vi "Measurement.TestLauncher.vi"() -> ()   [LabVIEW 2017]
uses:
  Typedefs/Measurement.Type--Enum.ctl
  Measurement.Free/Measurement.Free.lvclass
  D:/upwork/Laser Measurement Tool/Laser/project/Subsystems/Measurement/Measurement.lvclass
  Measurement.Free.UI/Measurement.Free.UI.lvclass
  D:/upwork/Laser Measurement Tool/Laser/project/Subsystems/Measurement.UI/Measurement.UI.lvclass
  Measurement.Free/Typedefs/Configuration--Cluster.ctl
  Measurement.Free/Typedefs/Configuration.Hardware--Cluster.ctl
  Typedefs/Configuration.SMU--Cluster.ctl
  SMU/Typedefs/Configuration--Cluster.ctl
  Typedefs/Configuration.LIA--Cluster.ctl
  LIA/Typedefs/Configuration--Cluster.ctl
  Typedefs/Configuration.OPM--Cluster.ctl
  OPM/Typedefs/Configuration--Cluster.ctl
  Typedefs/Configuration.OPA--Cluster.ctl
  OPA/Typedefs/Configuration--Cluster.ctl
  Measurement.lvclass
  OPA/OPA.lvclass
  OPM/OPM.lvclass
  LIA/LIA.lvclass
  SMU/SMU.lvclass
  OPA.OrpheusHP/OPA.OrpheusHP.lvclass
  OPM.ThorlabsPM400/OPM.ThorlabsPM400.lvclass
panel:
  in  "Close":bool
  out "Measurements Tree":string(tree) caption="Chart A"
  in  "Add":bool
  in  "Remove":bool
  in  "Stop":bool
  in  "Start":bool
  in  "Measurement Parameters":T1(tab)
  in  "Accumulation":dbl=10.0 caption="Numeric"
  in  "Delay Time":dbl[unit]=0.5
  in  "Integration Time":dbl[unit]=3.0
  in  "Scan Resolution":dbl[unit]=2e-08
  in  "Number of Points":dbl caption="Numeric"
  in  "Stop Wavelength":dbl[unit]=1.0000000000000002e-06
  in  "Start Wavelength":dbl[unit]=6.000000000000001e-07
  in  "Sync":bool
  in  "Save":bool
  in  "Hardware Parameters":enum32{"Free"}(tab)
  in  "OPA Refresh List":bool
  in  "OPA Serial Number":string(combo)
  in  "OPM Refresh List":bool
  in  "OPM Simulated":bool
  in  "OPM Resource Name":string(combo)="USB0::0x1313::0x8075::P5001221::INSTR"
  in  "SMU Channel":string(combo)="A"
  in  "SMU Simulated":bool
  in  "SMU VISA Resource Name":refnum<visa-resource-name>="GPIB0::26::INSTR"
  in  "LIA Simulated":bool
  in  "LIA VISA Resource Name":refnum<visa-resource-name>="GPIB0::8::INSTR"
  out "Status":string
  out "Progress":u8(slide) scale=0.0..100.0
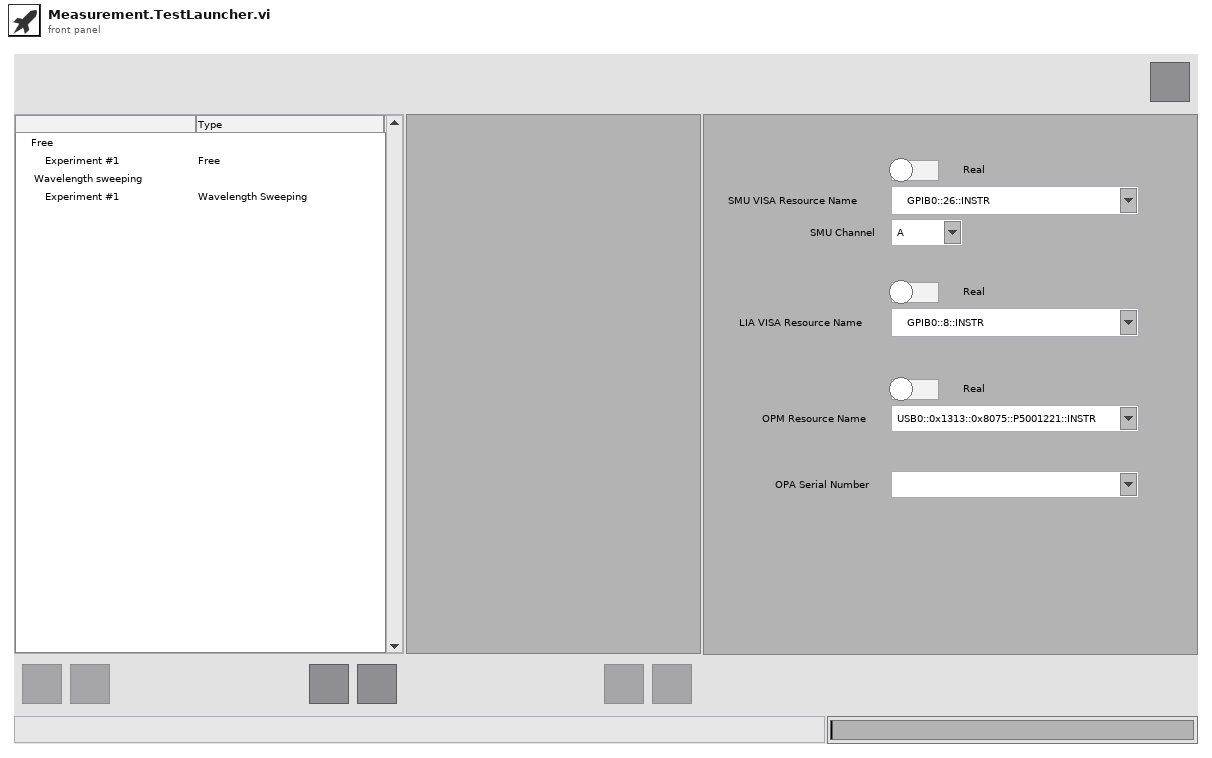
[diagram p1: front panel]
types:
  T1 = enum32{"Free", "Wavelength Sweeping", "Photocurrent mapping"}
  T2 = typedef "Measurement.lvclass/Measurement.Type--Enum.ctl" = enum16{"Free", "I/V Curve", "Wavelength sweeping", "Photocurrent mapping"}
  T3 = enum16{"Free", "I/V Curve", "Wavelength sweeping", "Photocurrent mapping"}
  T4 = enum8{"Enabled", "Disabled", "Disabled and Grayed Out"}
  T5 = typedef "LVPoint32TypeDef.ctl" = cluster{"Horizontal":i32, "Vertical":i32}
  T6 = typedef "Measurement.lvclass/Configuration.OPA--Cluster.ctl" = cluster{"Enable":bool, "OPA Model":string, "Configuration":T7}
  T7 = typedef "OPA.lvclass/Configuration--Cluster.ctl" = cluster{"Serial Number":string}
  T8 = typedef "Measurement.lvclass/Configuration.OPM--Cluster.ctl" = cluster{"Enable":bool, "OPM Model":string, "Configuration":T9}
  T9 = typedef "OPM.lvclass/Configuration--Cluster.ctl" = cluster{"VISA Resource":string}
  T10 = typedef "Measurement.lvclass/Configuration.LIA--Cluster.ctl" = cluster{"Enable":bool, "LIA Model":string, "Configuration":T11}
  T11 = typedef "LIA.lvclass/Configuration--Cluster.ctl" = cluster{"VISA Resource":string}
  T12 = typedef "Measurement.lvclass/Configuration.SMU--Cluster.ctl" = cluster{"Enable":bool, "SMU Model":string, "Configuration":T13}
  T13 = typedef "SMU.lvclass/Configuration--Cluster.ctl" = cluster{"VISA Resource":string, "Channel":string}
  T14 = typedef "Measurement.Free.lvclass/Configuration--Cluster.ctl" = cluster{"Measurement.Type":enum16{"Free", "I/V Curve", "Wavelength sweeping", "Photocurrent mapping"}, "Hardware":T15}
  T15 = typedef "Measurement.Free.lvclass/Configuration.Hardware--Cluster.ctl" = cluster{"SMU":T12, "LIA":T10, "OPM":T8, "OPA":T6}
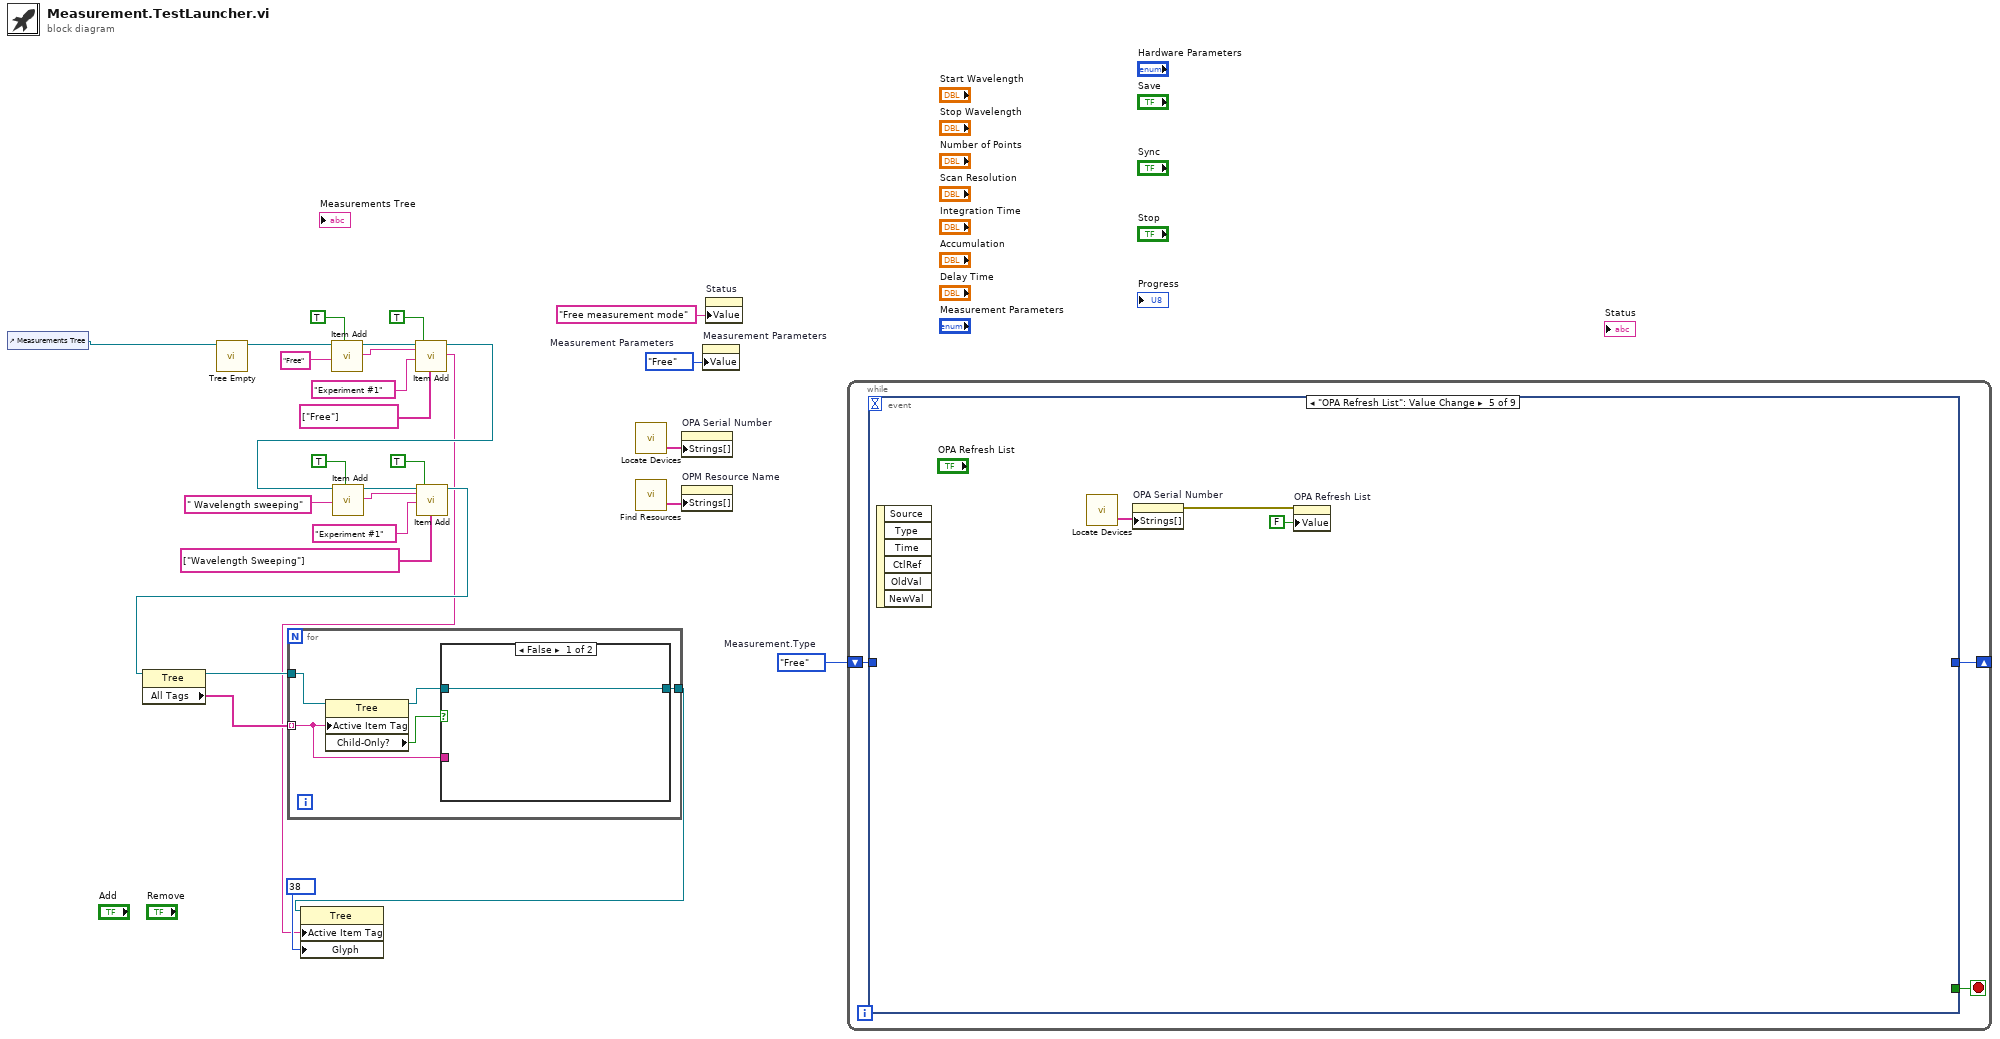
[diagram p0: block diagram]
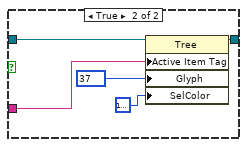
[diagram p2: hidden frame]
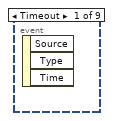
[diagram p3: hidden frame]
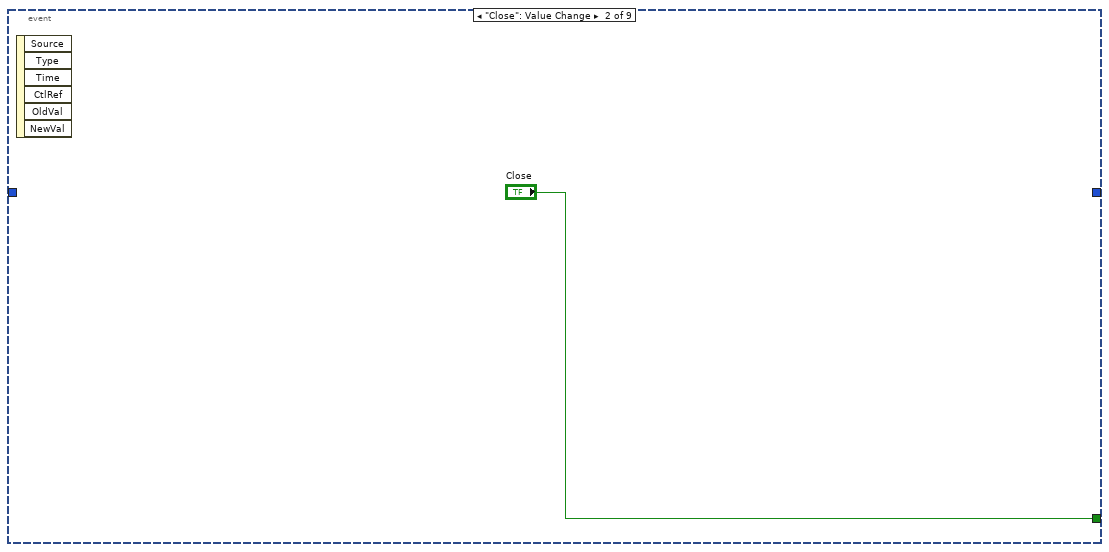
[diagram p4: hidden frame]
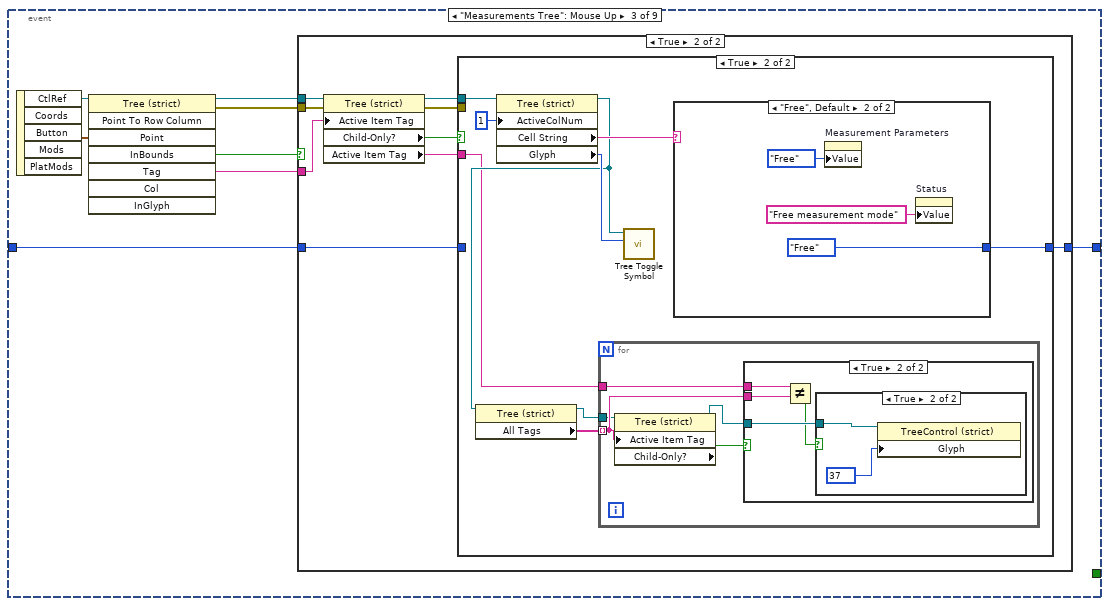
[diagram p5: hidden frame]
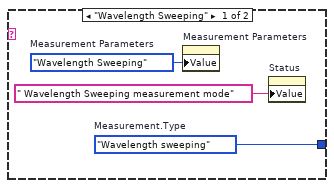
[diagram p10: hidden frame]
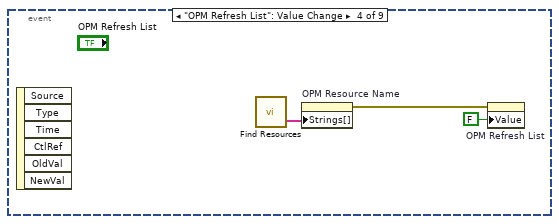
[diagram p11: hidden frame]
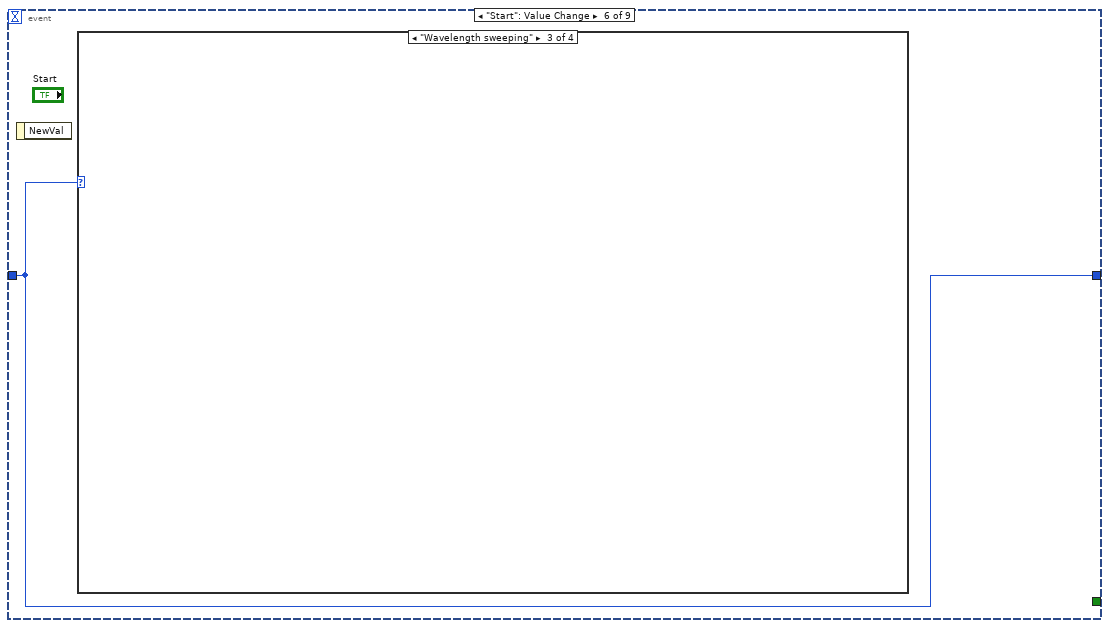
[diagram p12: hidden frame]
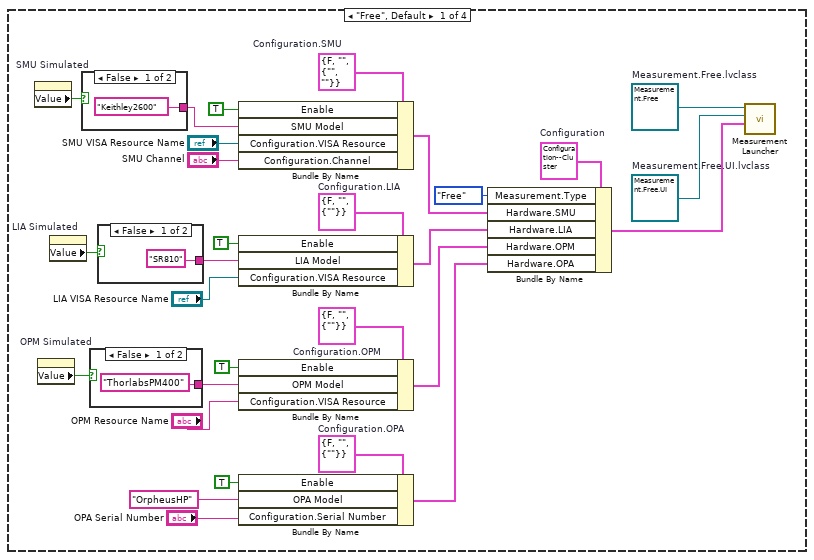
[diagram p13: hidden frame]
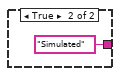
[diagram p14: hidden frame]
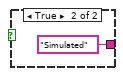
[diagram p15: hidden frame]
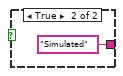
[diagram p16: hidden frame]
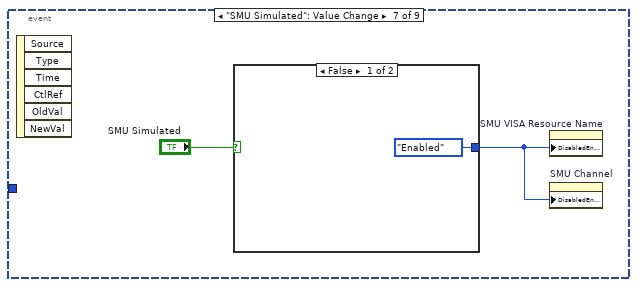
[diagram p19: hidden frame]
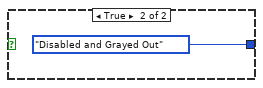
[diagram p20: hidden frame]
diagram:
  w2 = T1."Free"  # Measurement Parameters
  w28 = Measurement.Type--Enum."Free"  # Measurement.Type
  n1 = control-ref of="Measurements Tree"() -> (w10:refnum<vi>)
  n2 = call <instrlib>:"Tree Empty.vi"("Tree Reference In"=w10) -> ("Tree Reference Out"=w18:refnum<vi>)  [unwired: 16 in, 2 out]
  n3 = call <instrlib>:"Item Add.vi"("Tree Reference In"=w18, "New Text Value"="Free", "Make Top Level Item"=TRUE) -> ("Tree Reference Out"=w19:refnum<vi>, "Created Tag"=w23:string)  [unwired: 14 in, 1 out]
  n4 = call <instrlib>:"Item Add.vi"("Tree Reference In"=w19, "Parent Tag (Current)"=w23, "New Text Value"="Experiment #1", "Child Only?"=TRUE, "Column Text{#1 and greater}(empty)"=string[] ["Free"]) -> ("Tree Reference Out"=w6:refnum<vi>, "Created Tag"=w3:string)  [unwired: 12 in, 1 out]
  n5 = call <instrlib>:"Item Add.vi"("Tree Reference In"=w6, "New Text Value"=" Wavelength sweeping", "Make Top Level Item"=TRUE) -> ("Tree Reference Out"=w17:refnum<vi>, "Created Tag"=w13:string)  [unwired: 14 in, 1 out]
  n6 = call <instrlib>:"Item Add.vi"("Tree Reference In"=w17, "Parent Tag (Current)"=w13, "New Text Value"="Experiment #1", "Child Only?"=TRUE, "Column Text{#1 and greater}(empty)"=string[] ["Wavelength Sweeping"]) -> ("Tree Reference Out"=w7:refnum<vi>)  [unwired: 12 in, 2 out]
  n7 = property on="Property Node" class="Tree"(reference=w7) -> (reference out=w8:refnum<vi>, "All Tags"=w9:string[])  [unwired: 1 in, 1 out]
  n8 = for {
    tunnel: w9 -> [w30] mode=indexing
    tunnel: w8 -> [w33]
    tunnel: [w29] -> w4
    n9 = property class="Tree"(reference=w33, "Active Item Tag"=w30) -> (reference out=w32:refnum<vi>, "Child-Only?"=w31:bool)  [unwired: 1 in, 1 out]
    n10 = case shown="False" w31 {
      tunnel: w32 -> [w34 w37]
      tunnel: w30 -> [_ w36]
      tunnel: [w34 w35] -> w29
      frame False {
      }
      frame True {
        n11 = property class="Tree"(reference=w37, "Active Item Tag"=w36, "Glyph"=37, "SelColor"=u32 16777216) -> (reference out=w35:refnum<vi>)  [unwired: 1 in, 1 out]
      }
    }
  }
  n12 = property class="Tree"(reference=w4, "Active Item Tag"=w3, "Glyph"=38) -> ()  [unwired: 1 in, 2 out]
  n13 = call "Locate Devices.vi"() -> ("Serial Numbers"=w27:string[])  [unwired: 2 in, 1 out]
  n14 = call "Find Resources.vi"() -> ("Resource Names"=w26:string[])  [unwired: 2 in, 1 out]
  n15 = property on="OPA Serial Number" class="CmbBox"("Strings[]"=w27) -> ()  [unwired: 2 in, 2 out]
  n16 = property on="OPM Resource Name" class="CmbBox"("Strings[]"=w26) -> ()  [unwired: 2 in, 2 out]
  n17 = property on="Measurement Parameters" class="TabCtl (strict)"("Value"=w2) -> ()  [unwired: 2 in, 2 out]
  n18 = property on="Status" class="Str"("Value"="Free measurement mode" ("Status")) -> ()  [unwired: 2 in, 2 out]
  n19 = while {
    shift-right: [w40] -> _
    shift-left: w28 -> [w41]
    stop <- w42 stop-if-true
    n20 = event shown="[4] \"OPA Refresh List\": Value Change" {
      selector: _ -> [_ _ _ _ _ _ _ _ _]
      dyn-events: _ -> [_ _ _ _ _ _ _ _ _]
      timeout: _ -> [_ _ _ _ _ _ _ _ _]
      tunnel: [_ "Close" _ _ _ _ _ _ _] -> w42
      tunnel: w41 -> [_ _ w44 _ _ w95 _ _ _]
      tunnel: [_ _ w45 _ _ w95 _ _ _] -> w40
      event Timeout {
        n21 = event-data() -> ()  [unwired: 1 in, 3 out]
      }
      event "Close": Value Change {
        n22 = event-data() -> ()  [unwired: 1 in, 6 out]
      }
      event "Measurements Tree": Mouse Up {
        n23 = event-data() -> ("CtlRef"=w51:refnum<vi>, "Coords"=w50:T5)  [unwired: 1 in, 3 out]
        n24 = invoke class="Tree (strict)" method="Point To Row Column"(reference=w51, "Point"=w50) -> (reference out=w49:refnum<vi>, error out=w48:errorcluster, "InBounds"=w46:bool, "Tag"=w47:string)  [unwired: 6 in, 4 out]
        n25 = case shown="True" w46 {
          tunnel: w49 -> [_ w61]
          tunnel: w48 -> [_ w56]
          tunnel: w47 -> [_ w60]
          tunnel: [w52 w54] -> w45
          tunnel: w44 -> [w52 w53]
          frame False {
          }
          frame True {
            n26 = property class="Tree (strict)"(reference=w61, error in=w56, "Active Item Tag"=w60) -> (reference out=w57:refnum<vi>, error out=w55:errorcluster, "Child-Only?"=w59:bool, "Active Item Tag"=w58:string)
            n27 = case shown="True" w59 {
              tunnel: w58 -> [_ w64]
              tunnel: w57 -> [_ w71]
              tunnel: w55 -> [_ _]
              tunnel: [w62 w68] -> w54
              tunnel: w53 -> [w62 _]
              frame False {
              }
              frame True {
                n28 = property class="Tree (strict)"(reference=w71, "ActiveColNum"=1 ("Active Cell:Active Column Number")) -> (reference out=w66:refnum<vi>, "Cell String"=w69:string, "Glyph"=w67:i32)  [unwired: 1 in, 1 out]
                n29 = property class="Tree (strict)"(reference=w66) -> (reference out=w63:refnum<vi>, "All Tags"=w65:string[])  [unwired: 1 in, 1 out]
                n30 = for {
                  tunnel: w65 -> [w74] mode=indexing
                  tunnel: w64 -> [w75]
                  tunnel: w63 -> [w72]
                  n31 = property class="Tree (strict)"(reference=w72, "Active Item Tag"=w74) -> (reference out=w73:refnum<vi>, "Child-Only?"=w76:bool)  [unwired: 1 in, 1 out]
                  n32 = case shown="True" w76 {
                    tunnel: w75 -> [_ w80]
                    tunnel: w74 -> [_ w79]
                    tunnel: w73 -> [_ w78]
                    frame False {
                    }
                    frame True {
                      n33 = Not Equal?(x=w80, y=w79) -> (x != y?=w77:bool)
                      n34 = case shown="True" w77 {
                        tunnel: w78 -> [_ w82]
                        frame False {
                        }
                        frame True {
                          n35 = property class="TreeControl (strict)"(reference=w82, "Glyph"=37) -> ()  [unwired: 1 in, 2 out]
                        }
                      }
                    }
                  }
                }
                n36 = call "Tree Toggle Symbol.vi"("Symbol"=w67, "TreeControl in"=w66) -> ()  [unwired: 7 in, 3 out]
                n37 = case shown="\"Free\", Default" w69 {
                  tunnel: [w84 Measurement.Type--Enum."Free" ("Measurement.Type")] -> w68
                  frame "Wavelength Sweeping" {
                    w84 = Measurement.Type--Enum."Wavelength sweeping"  # Measurement.Type
                    w85 = T1."Wavelength Sweeping"  # Measurement Parameters
                    n38 = property on="Measurement Parameters" class="TabCtl (strict)"("Value"=w85) -> ()  [unwired: 2 in, 2 out]
                    n39 = property on="Status" class="Str"("Value"=" Wavelength Sweeping measurement mode" ("Status")) -> ()  [unwired: 2 in, 2 out]
                  }
                  frame "Free", Default {
                    n40 = property on="Measurement Parameters" class="TabCtl (strict)"("Value"=T1."Free" ("Measurement Parameters")) -> ()  [unwired: 2 in, 2 out]
                    n41 = property on="Status" class="Str"("Value"="Free measurement mode" ("Status")) -> ()  [unwired: 2 in, 2 out]
                  }
                }
              }
            }
          }
        }
      }
      event "OPM Refresh List": Value Change {
        n42 = event-data() -> ()  [unwired: 1 in, 6 out]
        n43 = call "Find Resources.vi"() -> ("Resource Names"=w91:string[])  [unwired: 2 in, 1 out]
        n44 = property on="OPM Resource Name" class="CmbBox"("Strings[]"=w91) -> (error out=w90:errorcluster)  [unwired: 2 in, 1 out]
        n45 = property on="OPM Refresh List" class="Bool (strict)"(error in=w90, "Value"=FALSE ("OPM Refresh List")) -> ()  [unwired: 1 in, 2 out]
      }
      event "OPA Refresh List": Value Change {
        n46 = event-data() -> ()  [unwired: 1 in, 6 out]
        n47 = call "Locate Devices.vi"() -> ("Serial Numbers"=w94:string[])  [unwired: 2 in, 1 out]
        n48 = property on="OPA Serial Number" class="CmbBox"("Strings[]"=w94) -> (error out=w93:errorcluster)  [unwired: 2 in, 1 out]
        n49 = property on="OPA Refresh List" class="Bool (strict)"(error in=w93, "Value"=FALSE ("OPA Refresh List")) -> ()  [unwired: 1 in, 2 out]
      }
      event "Start": Value Change {
        n50 = event-data() -> ()  [unwired: 1 in, 1 out]
        n51 = case shown="\"Wavelength sweeping\"" w95 {
          frame "Free", Default {
            w99 = T6 {"Enable"=FALSE, "OPA Model"="", "Configuration"={"Serial Number"=""}}  # Configuration.OPA
            w106 = T8 {"Enable"=FALSE, "OPM Model"="", "Configuration"={"VISA Resource"=""}}  # Configuration.OPM
            w112 = T10 {"Enable"=FALSE, "LIA Model"="", "Configuration"={"VISA Resource"=""}}  # Configuration.LIA
            w121 = T12 {"Enable"=FALSE, "SMU Model"="", "Configuration"={"VISA Resource"="", "Channel"=""}}  # Configuration.SMU
            w122 = T14 {"Measurement.Type"=enum."Free", "Hardware"={"SMU"={"Enable"=FALSE, "SMU Model"="", "Configuration"={"VISA Resource"="", "Channel"=""}}, "LIA"={"Enable"=FALSE, "LIA Model"="", "Configuration"={"VISA Resource"=""}}, "OPM"={"Enable"=FALSE, "OPM Model"="", "Configuration"={"VISA Resource"=""}}, "OPA"={"Enable"=FALSE, "OPA Model"="", "Configuration"={"Serial Number"=""}}}}  # Configuration
            w123 = refnum<class "Measurement.Free.UI.lvclass"> refnum  # Measurement.Free.UI.lvclass
            w124 = refnum<class "Measurement.Free.lvclass"> refnum  # Measurement.Free.lvclass
            n52 = property on="SMU Simulated" class="Bool (strict)"() -> ("Value"=w113:bool)  [unwired: 2 in, 2 out]
            n53 = property on="OPM Simulated" class="Bool (strict)"() -> ("Value"=w104:bool)  [unwired: 2 in, 2 out]
            n54 = property on="LIA Simulated" class="Bool (strict)"() -> ("Value"=w109:bool)  [unwired: 2 in, 2 out]
            n55 = case shown="False" w113 {
              tunnel: ["Keithley2600" ("SMU Model") "Simulated" ("SMU Model")] -> w117
              frame False {
              }
              frame True {
              }
            }
            n56 = case shown="False" w104 {
              tunnel: ["ThorlabsPM400" ("SMU Model") "Simulated" ("SMU Model")] -> w103
              frame False {
              }
              frame True {
              }
            }
            n57 = case shown="False" w109 {
              tunnel: ["SR810" ("SMU Model") "Simulated" ("SMU Model")] -> w108
              frame False {
              }
              frame True {
              }
            }
            n58 = Bundle By Name(cluster=w121, "Enable"=TRUE, "SMU Model"=w117, "Configuration.VISA Resource"="SMU VISA Resource Name", "Configuration.Channel"="SMU Channel") -> (w116:T12)
            n59 = Bundle By Name(cluster=w112, "Enable"=TRUE, "LIA Model"=w108, "Configuration.VISA Resource"="LIA VISA Resource Name") -> (w111:T10)
            n60 = Bundle By Name(cluster=w106, "Enable"=TRUE, "OPM Model"=w103, "Configuration.VISA Resource"="OPM Resource Name") -> (w101:T8)
            n61 = Bundle By Name(cluster=w99, "Enable"=TRUE, "OPA Model"="OrpheusHP", "Configuration.Serial Number"="OPA Serial Number") -> (w100:T6)
            n62 = Bundle By Name(cluster=w122, "Measurement.Type"=T3."Free", "Hardware.SMU"=w116, "Hardware.LIA"=w111, "Hardware.OPM"=w101, "Hardware.OPA"=w100) -> (w114:T14)
            n63 = call "Measurement Launcher.vi"("Configuration"=w114, "Measurement.UI.lvclass"=w123, "Measurement.lvclass"=w124) -> ()  [unwired: 8 in, 1 out]
          }
          frame "I/V Curve" {
          }
          frame "Wavelength sweeping" {
          }
          frame "Photocurrent mapping" {
          }
        }
      }
      event "SMU Simulated": Value Change {
        n64 = event-data() -> ()  [unwired: 1 in, 6 out]
        n65 = case shown="False" "SMU Simulated" {
          tunnel: [T4."Enabled" ("Disabled") T4."Disabled and Grayed Out" ("Disabled")] -> w131
          frame False {
          }
          frame True {
          }
        }
        n66 = property on="SMU VISA Resource Name" class="VISAName"("DisabledEnum"=w131) -> ()  [unwired: 2 in, 2 out]
        n67 = property on="SMU Channel" class="CmbBox"("DisabledEnum"=w131) -> ()  [unwired: 2 in, 2 out]
      }
      event "LIA Simulated": Value Change {
        n68 = event-data() -> ()  [unwired: 1 in, 6 out]
        n69 = case shown="True" "LIA Simulated" {
          tunnel: [T4."Enabled" ("Disabled") T4."Disabled and Grayed Out" ("Disabled")] -> w135
          frame False {
          }
          frame True {
          }
        }
        n70 = property on="LIA VISA Resource Name" class="VISAName"("DisabledEnum"=w135) -> ()  [unwired: 2 in, 2 out]
      }
      event "OPM Simulated": Value Change {
        n71 = event-data() -> ()  [unwired: 1 in, 6 out]
        n72 = case shown="False" "OPM Simulated" {
          tunnel: [T4."Enabled" ("Disabled") T4."Disabled and Grayed Out" ("Disabled")] -> w139
          frame False {
          }
          frame True {
          }
        }
        n73 = property on="OPM Resource Name" class="CmbBox"("DisabledEnum"=w139) -> ()  [unwired: 2 in, 2 out]
      }
    }
  }
